vi "Paused Next State.vi"(8 "error in":errorcluster, 11 "Command":T2) -> (0 "error out":errorcluster, 3 "State":T1)   [LabVIEW 2013, in "Standard Engine Runtime.lvclass"]
uses:
  Standard Engine Runtime.lvclass
  Commands.ctl
  <vilib>/NI/Module Execution Interface/Engine Runtime/Execution States.ctl
  <vilib>/NI/Module Execution Interface/Engine Runtime/Engine Runtime Interface.lvclass
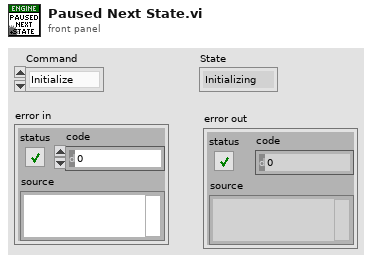
[diagram p1: front panel]
types:
  T1 = typedef "Engine Runtime Interface.lvclass/Execution States.ctl" = enum16{"Initializing", "Paused (Initialized)", "Running", "Set Safe Outputs", "Uninitializing", "Stopped (Uninitialized)", "Error (Uninitialized)", "Safe State (Uninitialized)", "Closed"}
  T2 = typedef "Standard Engine Runtime.lvclass/Commands.ctl" = enum16{"Initialize", "Start", "Pause", "Safe State", "Normal", "Stop", "Shutdown"}
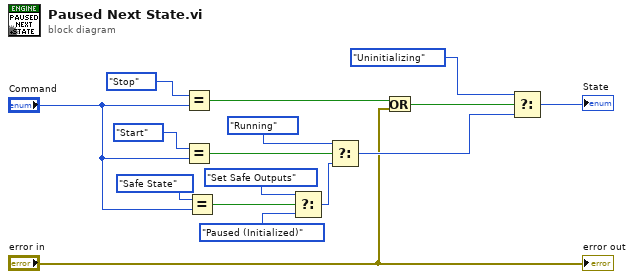
[diagram p0: block diagram]
diagram:
  n1 = Equal?(x=Commands."Stop" ("Commands"), y="Command") -> (x = y?=w11:bool)
  n2 = Equal?(x=Commands."Start" ("Commands"), y="Command") -> (x = y?=w8:bool)
  n3 = Equal?(x=Commands."Safe State" ("Commands"), y="Command") -> (x = y?=w4:bool)
  n4 = Select(t=Execution_States."Set Safe Outputs", s=w4, f=Execution_States."Paused (Initialized)" ("States")) -> (s? t:f=w2:T1)
  n5 = Select(t=Execution_States."Running" ("States"), s=w8, f=w2) -> (s? t:f=w10:T1)
  n6 = Or(x=w11, y="error in") -> (x .or. y?=w12:bool)
  n7 = Select(t=Execution_States."Uninitializing" ("States"), s=w12, f=w10) -> (s? t:f=→"State":T1)
  "error out" <- "error in"
